vi "Get Document Reference.vi"(8 "error in (no error)":errorcluster, 11 "ooDocument in":refnum<class "ooDocument.lvclass">) -> (0 "error out":errorcluster, 1 "Document":refnum<k24>, 3 "ooDocument out":refnum<class "ooDocument.lvclass">)   [LabVIEW 2009, in "ooDocument.lvclass"]
uses:
  ooDocument.lvclass
  C:/Projets/LAVAG/OpenOfficeRGT/AODL/DLLs/AODL.dll
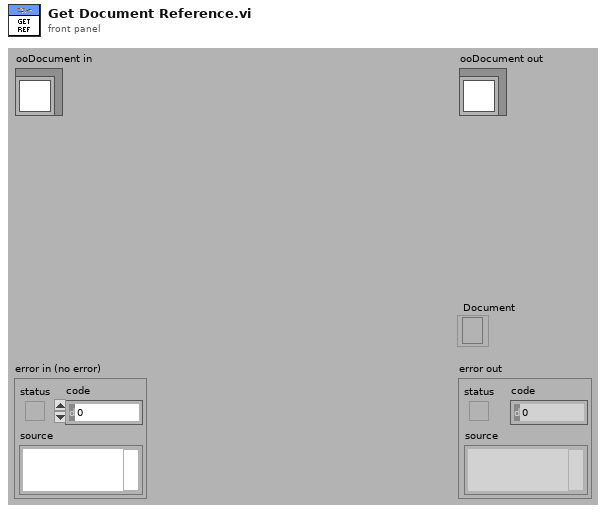
[diagram p1: front panel]
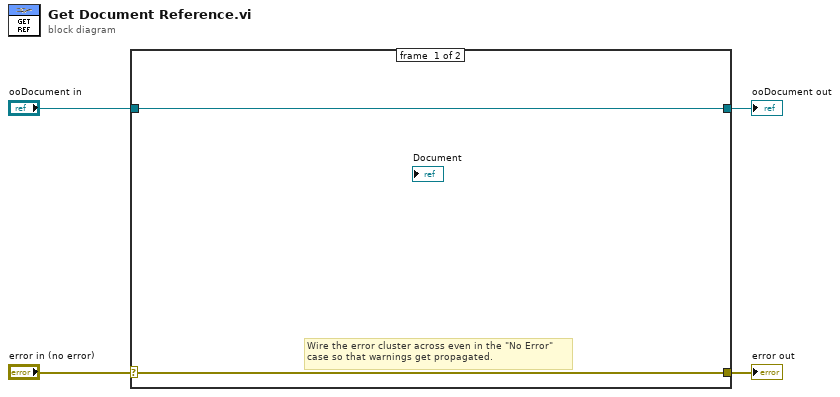
[diagram p0: block diagram]
diagram:
  n1 = case shown="No Error" "error in (no error)" {
    selector: "error in (no error)" -> [w5 w8]
    tunnel: [w5 w8] -> w3
    tunnel: [w6 w7] -> w1
    tunnel: "ooDocument in" -> [w6 w7]
    frame #0 {
      # "Wire the error cluster across even in the \"No Error\"\ncase so that warnings get propagated."
    }
    frame #1 {
    }
  }
  "error out" <- w3
  "ooDocument out" <- w1
